vi "Write Outgoing Bytes.vi"(8 "error in (no error)":errorcluster, 9 "timeout ms (2000)":i32=2000, 10 "Bytes":u8[](array[numeric]) format="%08b", 11 "Connection.LocalQueue":refnum<class "Connection.NetworkStream.lvclass">) -> (0 "error out":errorcluster, 1 "timeout":bool, 3 "Connection.LocalQueue":refnum<class "Connection.NetworkStream.lvclass">)   [LabVIEW 2013, in "Connection.NetworkQueue_GOSPL.lvlib" / "Connection.NetworkStream.lvclass"]
uses:
  Connection.NetworkStream/Connection.NetworkStream.lvclass
  Connection.NetworkStream/Connection.NetworkStream.lvclass/Connection.NetworkStream.ctl
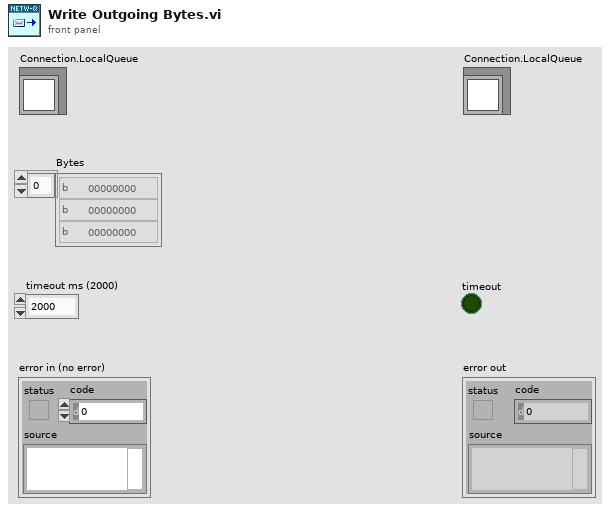
[diagram p1: front panel]
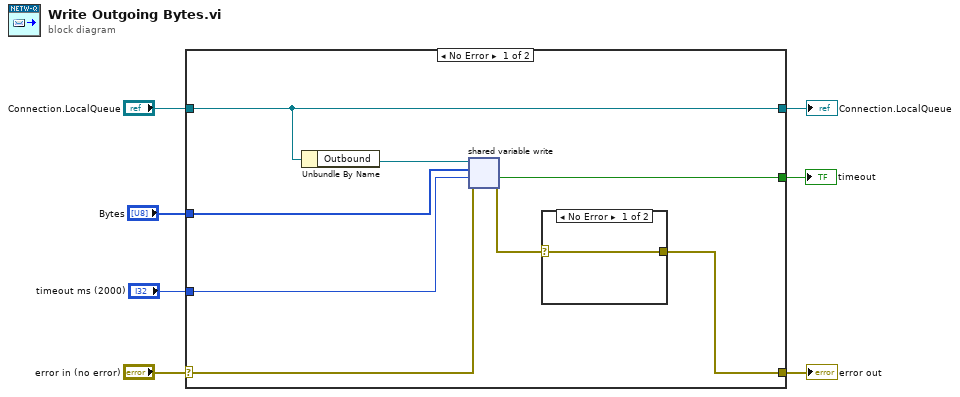
[diagram p0: block diagram]
diagram:
  n1 = case shown="No Error" "error in (no error)" {
    selector: "error in (no error)" -> [w10 w19]
    tunnel: [w14 w19] -> w6
    tunnel: [w15 w18] -> w4
    tunnel: "Connection.LocalQueue" -> [w15 w18]
    tunnel: "Bytes" -> [w12 _]
    tunnel: "timeout ms (2000)" -> [w11 _]
    tunnel: [w8 _] -> w1
    frame No Error {
      n2 = Unbundle By Name(w15) -> ("Outbound"=w13:refnum<k21>)
      n3 = shared-variable-write(w13, w10, w12, w11) -> (w9:errorcluster, w8:bool)  [unwired: 1 out]
      n4 = case shown="No Error" w9 {
        selector: w9 -> [w16 w17]
        tunnel: [w16 w17] -> w14
        frame No Error {
        }
        frame Error {
        }
      }
    }
    frame Error {
    }
  }
  "error out" <- w6
  "Connection.LocalQueue" <- w4
  "timeout" <- w1
